vi "Find Wire Terminals.vi"(11 "Wire":refnum<vi>) -> (1 "Sink Terminal":refnum<vi>, 2 "Source Terminal":refnum<vi>, 3 "Wire Dup":refnum<vi>)   [LabVIEW 2013, in "Abstract Param Writer.lvclass"]
doc: "Copyright (c) 2016 Sze Howe Koh\n\nThis Source Code Form is subject to the terms of the Mozilla Public License, v. 2.0. If a copy of the MPL was not distributed with this file, You can obtain one at http://mozilla.org/MPL/2.0/."
uses:
  Abstract Param Writer.lvclass
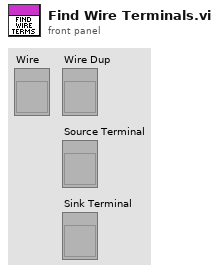
[diagram p1: front panel]
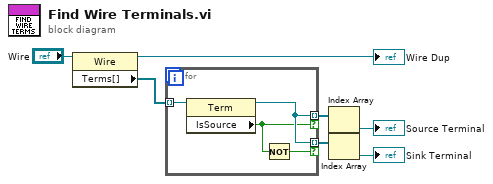
[diagram p0: block diagram]
diagram:
  n1 = property class="Wire"(reference="Wire") -> (reference out=→"Wire Dup":refnum<vi>, "Terms[]"=w7:refnum<vi>[])  [unwired: 1 in, 1 out]
  n2 = for {
    tunnel: w7 -> [w11] mode=indexing
    tunnel: [w10] -> w6 mode=indexing if=w9
    tunnel: [w10] -> w5 mode=indexing if=w8
    n3 = property class="Term"(reference=w11) -> (reference out=w10:refnum<vi>, "IsSource"=w9:bool)  [unwired: 1 in, 1 out]
    n4 = Not(x=w9) -> (.not. x?=w8:bool)
  }
  n5 = Index Array(array=w6) -> (element=→"Source Terminal":refnum<vi>)  [unwired: 1 in]
  n6 = Index Array(array=w5) -> (element=→"Sink Terminal":refnum<vi>)  [unwired: 1 in]
